vi "Wrap Ping Test.vi"(9 "PORT CONFIGURATION":T2(array[cluster]), 10 "DUT Info":T3, 11 "Interface Name":string) -> (0 "error out":errorcluster, 3 "PingResults":T1)   [LabVIEW 2026]
uses:
  DUT Info.ctl
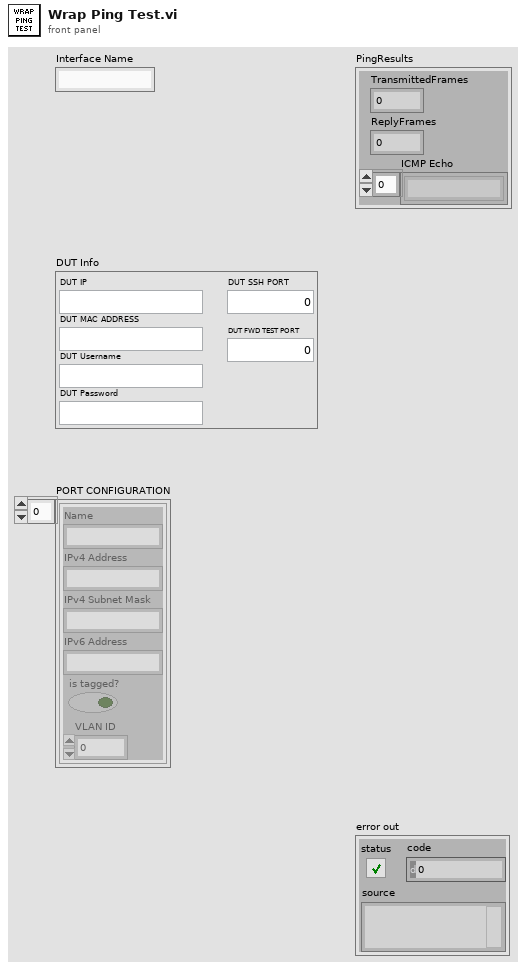
[diagram p1: front panel]
types:
  T1 = cluster{"TransmittedFrames":u32, "ReplyFrames":i32, "ICMP Echo ":string[]}
  T2 = cluster{"Name":string, "IPv4 Address":string, "IPv4 Subnet Mask":string, "IPv6 Address":string, "is tagged?":bool, "VLAN ID":u16}[]
  T3 = typedef "DUT Info.ctl" = cluster{"DUT IP":string, "DUT Username":string, "DUT Password":string, "DUT SSH PORT":u16, "DUT FWD TEST PORT":u16, "DUT MAC ADDRESS":string}
  T4 = typedef "DiagnosticModule.lvlib/ECUAddress.ctl" = cluster{"ECUIPv4Address":string, "SourceIPv4Address":string, "IsTagged":bool, "VLANID":u16}
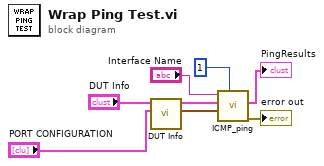
[diagram p0: block diagram]
diagram:
  n1 = call "DUT Info.vi"("PORT CONFIGURATION"="PORT CONFIGURATION", "DUT Info"="DUT Info") -> ("destination MAC address"=w5:cluster{u8, u8, u8, u8, u8, u8}, "Ping Addresses"=w2:T4[])  [unwired: 8 in]
  n2 = call "ICMP_ping.vi"("NumberOfRequestPerIP"=1, "destination MAC address"=w5, "PingAddresses"=w2, "ENETPort"="Interface Name") -> ("ErrorOut"=→"error out":errorcluster, "PingResults"=→"PingResults":T1)  [unwired: 5 in, 1 out]
